vi "Check Loop Error.vi"(9 "Ignore Errors":i32[](array[numeric]), 10 "error to process":errorcluster, 11 "Message Queue":refnum<queue>) -> (2 "Enqueued Error?":bool, 3 "dup Message Queue":refnum<queue>)   [LabVIEW 2024]
doc: "Check the 'error to process' to see if its code value matches any of the values in the 'Ignore Errors' array. If so, do nothing. If not, send an \"Error\" message containing the error data to the Message Handling Loop for further processing."
uses:
  Message Queue/Message Cluster.ctl
  Message Queue/Enqueue Message (Single).vi
  Message Queue/Message Queue.lvlib
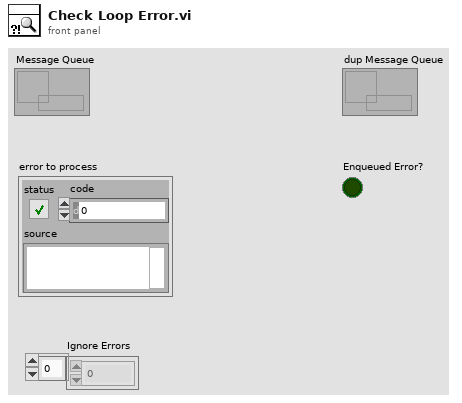
[diagram p1: front panel]
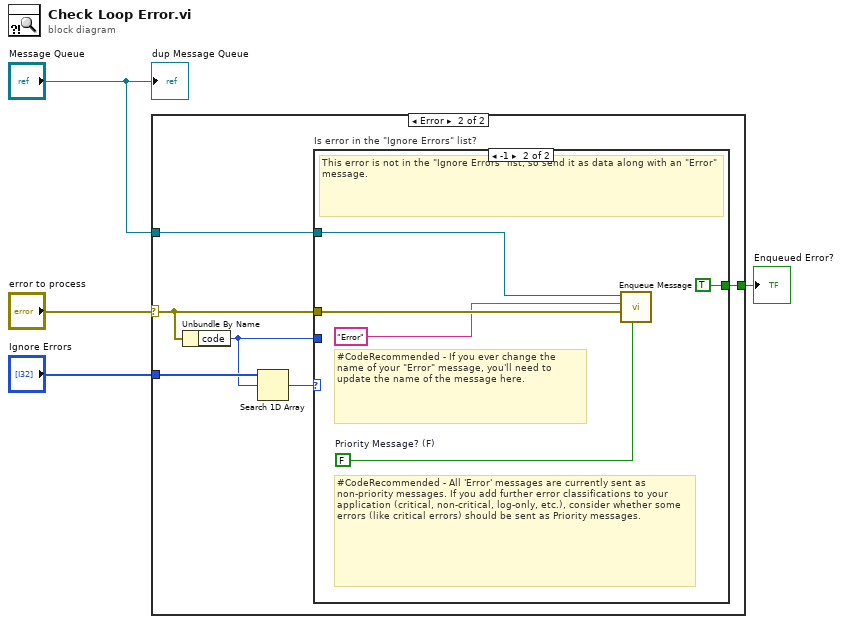
[diagram p0: block diagram]
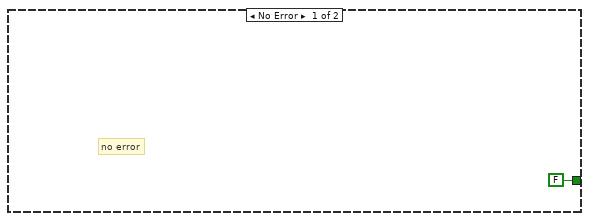
[diagram p2: hidden frame]
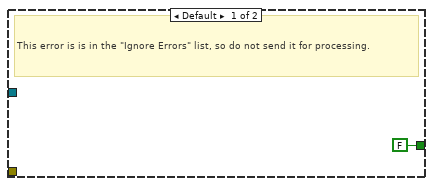
[diagram p3: hidden frame]
diagram:
  n1 = case shown="Error" "error to process" {
    selector: "error to process" -> [_ w7]
    tunnel: "Ignore Errors" -> [_ w11]
    tunnel: "Message Queue" -> [_ w9]
    tunnel: [FALSE ("Enqueued Error?") w6] -> w1
    frame No Error {
      # "no error"
    }
    frame Error {
      n2 = Unbundle By Name(w7) -> ("code"=w8:i32)
      n3 = Search 1D Array(1D array=w11, element=w8) -> (index of element=w10:i32)  [unwired: 1 in]
      n4 = case "Is error in the \"Ignore Errors\" list?" shown="-1" w10 {
        tunnel: w9 -> [_ w16]
        tunnel: w8 -> [_ _]
        tunnel: w7 -> [_ w17]
        tunnel: [FALSE ("Enqueued Error?") TRUE ("Enqueued Error?")] -> w6
        frame Default {
          # "This error is is in the \"Ignore Errors\" list, so do not send it for processing."
        }
        frame -1 {
          w14 = FALSE  # Priority Message? (F)
          # "#CodeRecommended - All 'Error' messages are currently sent as non-priority messages. If you add further error classifications to your application (critical, non-critical, log-only, etc.), consider whether some errors (like critical errors) should be sent as Priority messages."
          # "#CodeRecommended - If you ever change the name of your \"Error\" message, you'll need to update the name of the message here."
          # "This error is not in the \"Ignore Errors\" list, so send it as data along with an \"Error\" message."
          n5 = call-poly "Enqueue Message.vi"("Priority Message? (F)"=w14, "Message Data"=w17, "Message"="Error", "Message Queue"=w16) -> ()  [unwired: 6 in, 2 out]
        }
      }
    }
  }
  "Enqueued Error?" <- w1
  "dup Message Queue" <- "Message Queue"
